vi "Set Joint Commands.vi"(8 "error in (no error)":errorcluster, 9 "Close Gripper":bool, 10 "JointCommands":T1, 11 "Grips Robot in":refnum<class "Grips Robot.lvclass">) -> (0 "error out":errorcluster, 3 "Grips Robot out":refnum<class "Grips Robot.lvclass">)   [LabVIEW 2013, in "Grips Robot.lvclass"]
uses:
  Grips Robot.lvclass
  labview_ros/osrf_msgs/JointCommands.ctl
  labview_ros/std_msgs/Header.ctl
  Grips Robot.lvclass/Grips Robot.ctl
  Hardware Interface/Hardware Interface.lvclass/Hardware Interface.ctl
  Helpers/Get Element Index.vi
  <vilib>/addons/control/pid/pid.llb/PID (DBL).vi
  <vilib>/addons/control/pid/NI_PID_pid.lvlib
  Hardware Interface/Hardware Interface.lvclass
  Helpers/Helpers.lvlib
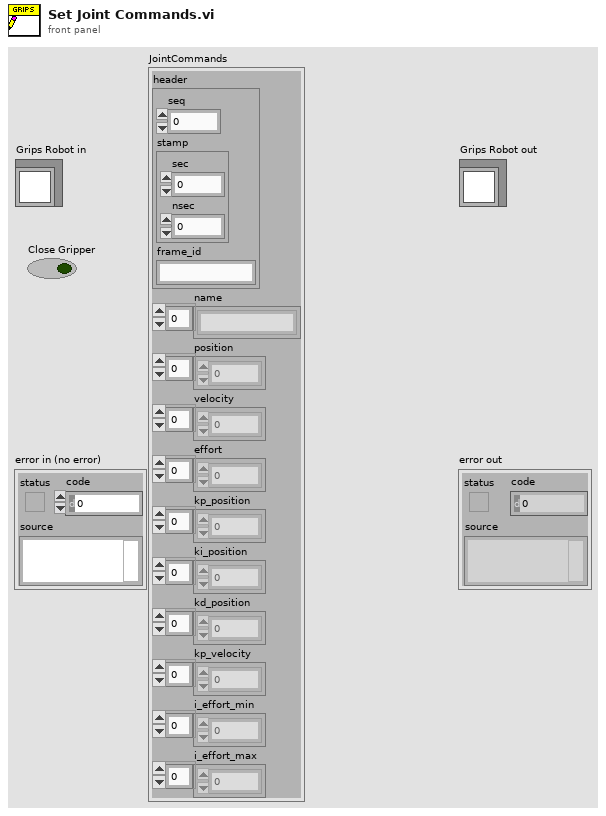
[diagram p1: front panel]
types:
  T1 = typedef "JointCommands.ctl" = cluster{"header":T2, "name":string[], "position":dbl[], "velocity":dbl[], "effort":dbl[], "kp_position":dbl[], "ki_position":dbl[], "kd_position":dbl[], "kp_velocity":dbl[], "i_effort_min":dbl[], "i_effort_max":dbl[]}
  T2 = typedef "Header.ctl" = cluster{"seq":u32, "stamp":cluster{"sec":i32, "nsec":i32}, "frame_id":string}
  T3 = cluster{"proportional gain (Kc)":dbl, "integral time (Ti, min)":dbl, "derivative time (Td, min)":dbl}
  T4 = typedef "Hardware Interface.lvclass/DblArrayWithName.ctl" = cluster{"name":string[], "value":dbl[]}
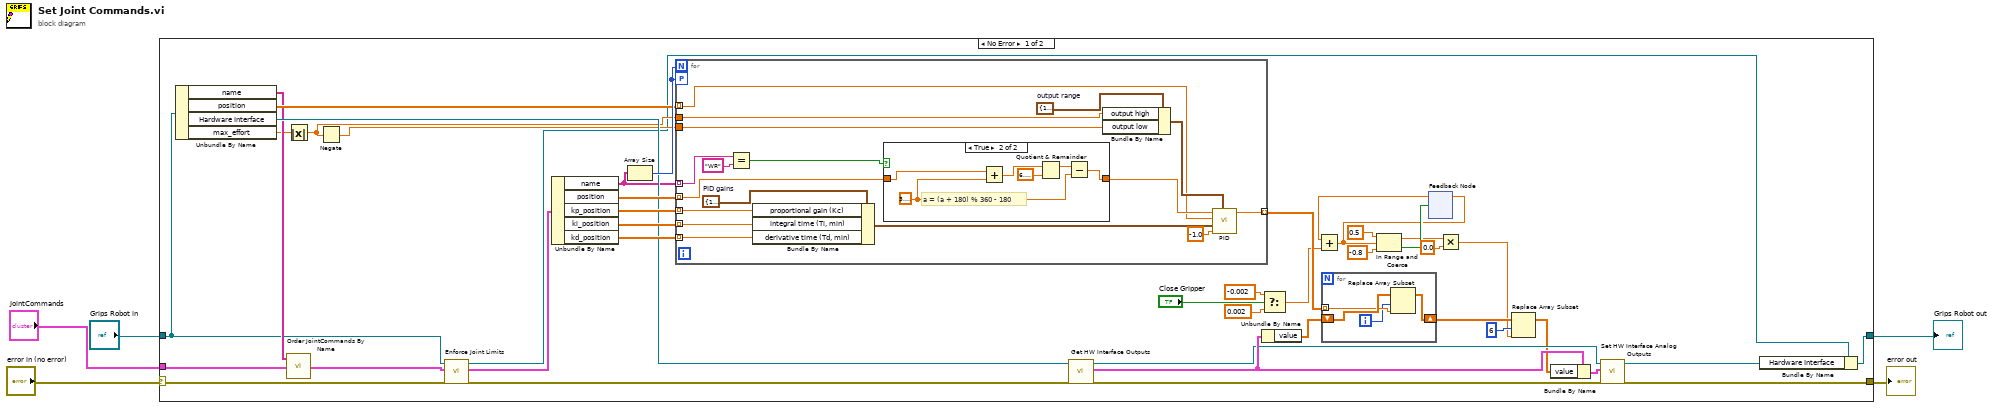
[diagram p0: block diagram]
diagram:
  n1 = case shown="No Error" "error in (no error)" {
    selector: "error in (no error)" -> [w9 w77]
    tunnel: [w41 w77] -> w4
    tunnel: [w48 w78] -> w2
    tunnel: "Grips Robot in" -> [w11 w78]
    tunnel: "JointCommands" -> [w32 _]
    frame No Error {
      n2 = Unbundle By Name(w11) -> ("name"=w31:string[], "position"=w36:dbl[], "Hardware Interface"=w35:refnum<class "Hardware Interface.lvclass">, "max_effort"=w30:dbl)
      n3 = Absolute Value(x=w30) -> (abs(x)=w29:dbl)
      n4 = call "Order JointCommands By Name.vi"("Ordered Joint Names"=w31, "JointCommands"=w32) -> ("Ordered JointCommands"=w14:T1)  [unwired: 7 in]
      n5 = Negate(x=w29) -> (-x=w28:dbl)
      n6 = call "Enforce Joint Limits.vi"("error in (no error)"=w9, "Joint Command"=w14, "Grips Robot in"=w11) -> ("error out"=w10:errorcluster, "Enforced Command"=w13:T1, "Grips Robot out"=w12:refnum<class "Grips Robot.lvclass">)  [unwired: 6 in]
      n7 = Unbundle By Name(w13) -> ("name"=w15:string[], "position"=w46:dbl[], "kp_position"=w45:dbl[], "ki_position"=w44:dbl[], "kd_position"=w43:dbl[])
      n8 = Array Size(array=w15) -> (size(s)=w47:i32)
      n9 = for {
        N: w47 -> [_]
        workers-P: w47 -> [_]
        tunnel: w36 -> [w53] mode=indexing
        tunnel: w46 -> [w56] mode=indexing
        tunnel: w45 -> [w67] mode=indexing
        tunnel: w44 -> [w66] mode=indexing
        tunnel: w43 -> [w65] mode=indexing
        tunnel: [w61] -> w33 mode=indexing
        tunnel: w29 -> [w60]
        tunnel: w28 -> [w59]
        tunnel: w15 -> [w58] mode=indexing
        w63 = cluster{"output high":dbl, "output low":dbl} {"output high"=100.0, "output low"=-100.0}  # output range
        w69 = T3 {"proportional gain (Kc)"=1.0, "integral time (Ti, min)"=0.01, "derivative time (Td, min)"=0.0}  # PID gains
        n10 = Equal?(x=w58, y="WR") -> (x = y?=w55:bool)
        n11 = Bundle By Name(cluster=w69, "proportional gain (Kc)"=w67, "integral time (Ti, min)"=w66, "derivative time (Td, min)"=w65) -> (w68:T3)
        n12 = case shown="True" w55 {
          tunnel: w56 -> [w70 w76]
          tunnel: [w70 w71] -> w54
          frame False {
          }
          frame True {
            w72 = 3.141592653589793
            # "a = (a + 180) % 360 - 180"
            n13 = Add(x=w76, y=w72) -> (x+y=w74:dbl)
            n14 = Quotient & Remainder(x=w74, y=6.283185307179586) -> (x-y*floor(x/y)=w73:dbl)  [unwired: 1 out]
            n15 = Subtract(x=w73, y=w72) -> (x-y=w71:dbl)
          }
        }
        n16 = Bundle By Name(cluster=w63, "output high"=w60, "output low"=w59) -> (w62:cluster{"output high":dbl, "output low":dbl})
        n17 = call-poly <vilib>:"PID.vi"("output range"=w62, "dt (s)"=-1.0, "PID gains"=w68, "process variable"=w53, "setpoint"=w54) -> ("output"=w61:dbl)  [unwired: 5 in, 1 out]
      }
      n18 = call "Get HW Interface Outputs.vi"("error in (no error)"=w10, "Hardware Interface in"=w35) -> ("error out"=w39:errorcluster, "Analog Outputs"=w38:T4, "Hardware Interface out"=w37:refnum<class "Hardware Interface.lvclass">)  [unwired: 6 in, 1 out]
      n19 = Unbundle By Name(w38) -> ("value"=w34:dbl[])
      n20 = Select(t=-0.002, s="Close Gripper", f=0.002) -> (s? t:f=w17:dbl)
      n21 = for {
        shift-right: [w50] -> w19
        shift-left: w34 -> [w52]
        tunnel: w33 -> [w51] mode=indexing
        i -> [w49]
        n22 = Replace Array Subset(array=w52, new element=w51, index=w49) -> (w50:dbl[])
      }
      n23 = feedback #1() -> (w23:dbl)  [unwired: 1 in]
      n24 = Add(x=w23, y=w17) -> (x+y=w20:dbl)
      n25 = In Range and Coerce(upper limit=0.5, x=w20, lower limit=-0.8) -> (coerced(x)=w8:dbl, In Range?=w22:bool)
      n26 = feedback-in #1(w20, w22) -> ()
      n27 = Multiply(x=w8, y=0.0) -> (x*y=w7:dbl)
      n28 = Replace Array Subset(array=w19, new element=w7, index=6) -> (w18:dbl[])
      n29 = Bundle By Name(cluster=w38, "value"=w18) -> (w40:T4)
      n30 = call "Set HW Interface Analog Outputs.vi"("error in (no error)"=w39, "Analog Outputs"=w40, "Hardware Interface in"=w37) -> ("error out"=w41:errorcluster, "Hardware Interface out"=w42:refnum<class "Hardware Interface.lvclass">)  [unwired: 7 in]
      n31 = Bundle By Name(cluster=w12, "Hardware Interface"=w42) -> (w48:refnum<class "Grips Robot.lvclass">)
    }
    frame Error {
    }
  }
  "error out" <- w4
  "Grips Robot out" <- w2
